vi "Read App Config_Machine.vi"(11 "App Config Path":path) -> (2 "Cal Files Path":path, 3 "Registered Systems":T1[](array[typedef]))   [LabVIEW 2013]
uses:
  Type Defs/Registered Machines.ctl
  <vilib>/Utility/config.llb/Read Key (Path).vi
  <vilib>/Utility/config.llb/Read Key (String).vi
  <vilib>/Utility/config.llb/Write Key (Path).vi
  <vilib>/Utility/config.llb/NI_LVConfig.lvlib
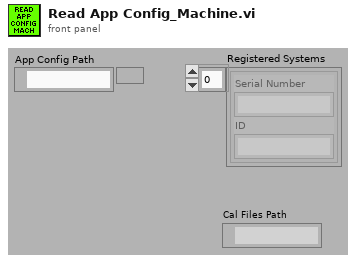
[diagram p1: front panel]
types:
  T1 = typedef "Registered Machines.ctl" = cluster{"Serial Number":string, "ID":string}
  T2 = typedef "NI_LVConfig.lvlib/Config Data RefNum.ctl" = refnum<k1>
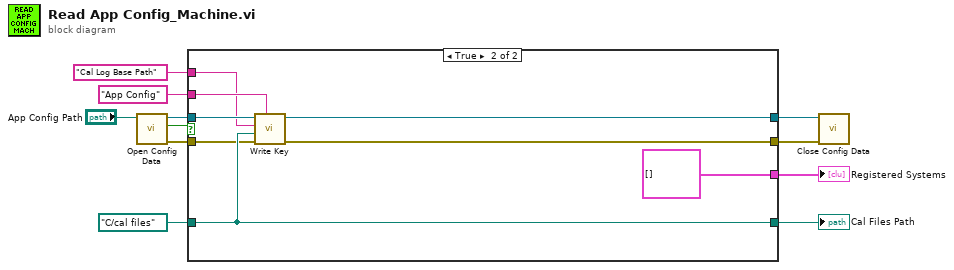
[diagram p0: block diagram]
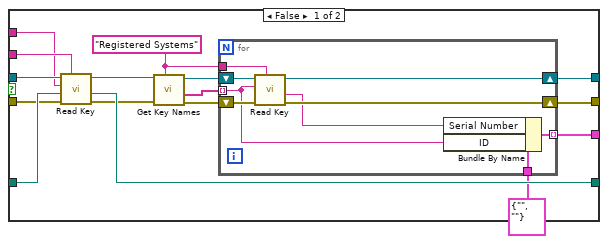
[diagram p2: hidden frame]
diagram:
  n1 = call <vilib>:"Open Config Data.vi"("configuration file path"="App Config Path") -> ("error out"=w6:errorcluster, "file created?"=w10:bool, "refnum"=w7:T2)  [unwired: 8 in]
  n2 = case shown="True" w10 {
    tunnel: w6 -> [w25 w42]
    tunnel: w7 -> [w26 w43]
    tunnel: [w17 w41] -> w8
    tunnel: [w18 w40] -> w9
    tunnel: path "C:/cal files" ("default value") -> [w27 w44]
    tunnel: [w24 w44] -> w4
    tunnel: "App Config" ("section") -> [w16 w39]
    tunnel: "Cal Log Base Path" ("section") -> [w15 w38]
    tunnel: [w12 T1[] [] ("Registered Systems")] -> w1
    frame False {
      w20 = "Registered Systems" ("section")
      n3 = call-poly <vilib>:"Read Key.vi"("section"=w16, "error in (no error)"=w25, "default value"=w27, "key"=w15, "refnum"=w26) -> ("error out"=w19:errorcluster, "value"=w24:path, "refnum out"=w14:T2)  [unwired: 3 in, 1 out]
      n4 = call <vilib>:"Get Key Names.vi"("section"=w20, "error in (no error)"=w19, "refnum"=w14) -> ("error out"=w22:errorcluster, "key names"=w21:string[], "refnum out"=w23:T2)  [unwired: 5 in, 1 out]
      n5 = for {
        tunnel: w20 -> [w36]
        tunnel: w21 -> [w30] mode=indexing
        shift-right: [w34] -> w17
        shift-left: w22 -> [w35]
        shift-right: [w32] -> w18
        shift-left: w23 -> [w33]
        tunnel: T1 {"Serial Number"="", "ID"=""} ("Registered System") -> [w31]
        tunnel: [w29] -> w12 mode=indexing
        n6 = call-poly <vilib>:"Read Key.vi"("section"=w36, "error in (no error)"=w35, "key"=w30, "refnum"=w33) -> ("error out"=w34:errorcluster, "value"=w28:string, "refnum out"=w32:T2)  [unwired: 4 in, 1 out]
        n7 = Bundle By Name(cluster=w31, "Serial Number"=w28, "ID"=w30) -> (w29:T1)
      }
    }
    frame True {
      n8 = call-poly <vilib>:"Write Key.vi"("section"=w39, "error in (no error)"=w42, "value"=w44, "key"=w38, "refnum"=w43) -> ("error out"=w41:errorcluster, "refnum out"=w40:T2)  [unwired: 4 in, 1 out]
    }
  }
  "Cal Files Path" <- w4
  "Registered Systems" <- w1
  n9 = call <vilib>:"Close Config Data.vi"("error in (no error)"=w8, "refnum"=w9) -> ()  [unwired: 8 in, 2 out]
